vi "ConditionalPath.vi"(1 "Path in":path) -> (0 "Stop?":bool)   [LabVIEW 2020]
doc: "Displays the value of the path and allows conditional breakpoints."
panel:
  in  "Tab Control":enum32{"Data", "Condition"}(tab)
  out "Path out":path
  in  "Conditional String":string
  in  "Pause If:":u16(ring) items=["<None>", "Ends with", "Equals", "Starts with", "Contains", "Matches pattern"]
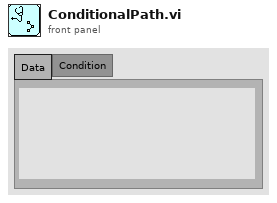
[diagram p1: front panel]
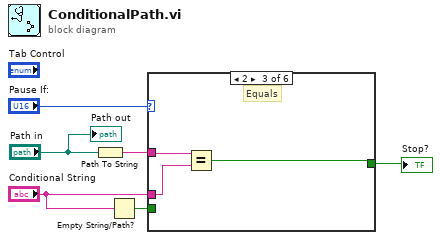
[diagram p0: block diagram]
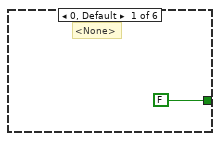
[diagram p2: hidden frame]
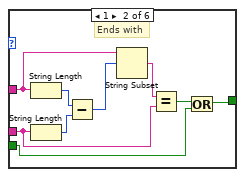
[diagram p3: hidden frame]
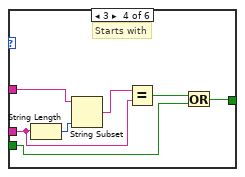
[diagram p4: hidden frame]
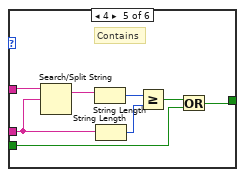
[diagram p5: hidden frame]
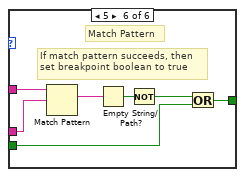
[diagram p6: hidden frame]
diagram:
  n1 = Path To String(path="Path in") -> (string=w2:string)
  n2 = Empty String/Path?(string/path="Conditional String") -> (empty?=w5:bool)
  n3 = case shown="2" "Pause If:" {
    tunnel: w2 -> [_ w12 w19 w23 w34 w41]
    tunnel: "Conditional String" -> [_ w10 w18 w20 w33 w40]
    tunnel: [FALSE w15 w17 w25 w27 w35] -> w4
    tunnel: w5 -> [_ w9 _ w21 w28 w37]
    frame 0, Default {
      # "<None>"
    }
    frame 1 {
      # "Ends with"
      n4 = String Length(string=w12) -> (length=w14:i32)
      n5 = String Length(string=w10) -> (length=w13:i32)
      n6 = Subtract(x=w14, y=w13) -> (x-y=w8:i32)
      n7 = String Subset(string=w12, offset (0)=w8) -> (substring=w11:string)  [unwired: 1 in]
      n8 = Equal?(x=w11, y=w10) -> (x = y?=w16:bool)
      n9 = Or(x=w16, y=w9) -> (x .or. y?=w15:bool)
    }
    frame 2 {
      # "Equals"
      n10 = Equal?(x=w19, y=w18) -> (x = y?=w17:bool)
    }
    frame 3 {
      # "Starts with"
      n11 = String Length(string=w20) -> (length=w24:i32)
      n12 = String Subset(string=w23, length (rest)=w24) -> (substring=w22:string)  [unwired: 1 in]
      n13 = Equal?(x=w22, y=w20) -> (x = y?=w26:bool)
      n14 = Or(x=w26, y=w21) -> (x .or. y?=w25:bool)
    }
    frame 4 {
      # "Contains"
      n15 = Search/Split String(string=w34, search string/char (-)=w33) -> (match + rest of string=w32:string)  [unwired: 1 in, 2 out]
      n16 = String Length(string=w32) -> (length=w31:i32)
      n17 = String Length(string=w33) -> (length=w30:i32)
      n18 = Greater Or Equal?(x=w31, y=w30) -> (x >= y?=w29:bool)
      n19 = Or(x=w29, y=w28) -> (x .or. y?=w27:bool)
    }
    frame 5 {
      # "Match Pattern"
      # "If match pattern succeeds, then\nset breakpoint boolean to true"
      n20 = Match Pattern(string=w41, regular expression=w40) -> (match substring=w39:string)  [unwired: 1 in, 3 out]
      n21 = Empty String/Path?(string/path=w39) -> (empty?=w38:bool)
      n22 = Not(x=w38) -> (.not. x?=w36:bool)
      n23 = Or(x=w36, y=w37) -> (x .or. y?=w35:bool)
    }
  }
  "Stop?" <- w4
  "Path out" <- "Path in"
